vi "Main VI task 2.vi"() -> ()   [LabVIEW 2024]
panel:
  in  "I_1":dbl
  out "I":dbl
  out "I_sh":dbl
  in  "R_sh":dbl
  in  "R_s":dbl
  in  "V":dbl
  out "I_0":dbl
  out "I_rs":dbl
  in  "G":dbl
  in  "N_s":dbl
  in  "V_OC":dbl
  out "I_ph":dbl
  in  "T":dbl
  in  "I_sc":dbl
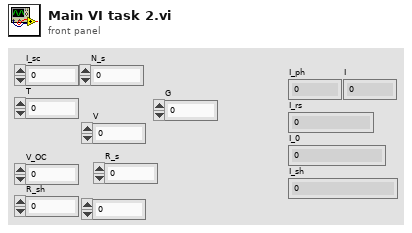
[diagram p1: front panel]
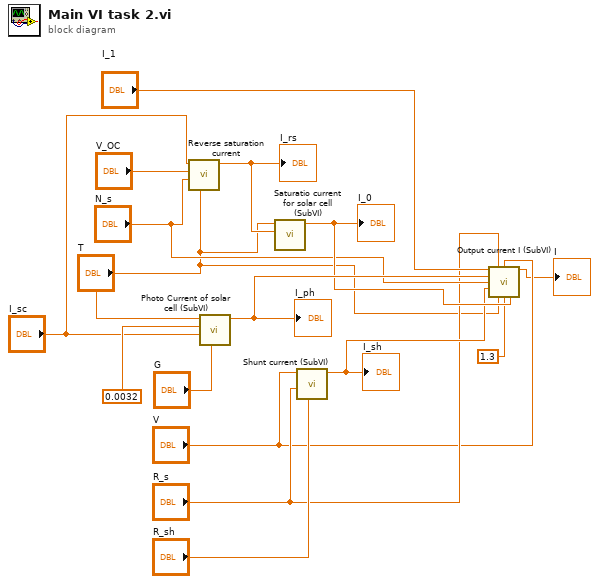
[diagram p0: block diagram]
diagram:
  n1 = call "Reverse saturation current.vi"("T"="T", "N_s"="N_s", "V_OC"="V_OC", "I_sc"="I_sc") -> ("I_rs"=w13:dbl)  [unwired: 7 in]
  "I_rs" <- w13
  n2 = call "Photo Current of solar cell (SubVI).vi"("G"="G", "I_sc"="I_sc", "k_i"=0.0032, "T"="T") -> ("I_ph"=w10:dbl)  [unwired: 7 in]
  "I_ph" <- w10
  n3 = call "Saturatio current for solar cell (SubVI).vi"("I_rs"=w13, "T"="T") -> ("I_0"=w9:dbl)  [unwired: 9 in]
  "I_0" <- w9
  n4 = call "Shunt current (SubVI).vi"("R_sh"="R_sh", "R_s"="R_s", "V"="V") -> ("I_sh"=w8:dbl)  [unwired: 8 in]
  "I_sh" <- w8
  n5 = call "Output current I (SubVI).vi"("I_1"="I_1", "R_s"="R_s", "V"="V", "I_ph"=w10, "N_s"="N_s", "I_sh"=w8, "T"="T", "n"=1.3, "I_0"=w9) -> ("I"=→"I":dbl)  [unwired: 6 in]
